vi "INI to JSON Test.vi"() -> ()   [LabVIEW 2017, in "JSONtext.lvlib"]
uses:
  JSONtext.lvlib
  support/quote and escape json string 2.vi
  <vilib>/JDP Science/JDP Science Common Utilities/JDP Utility.lvlib
panel:
  out "<JSON>":string
  out "String":string
  out "Array":string[](array[string])
  out "before substring":string
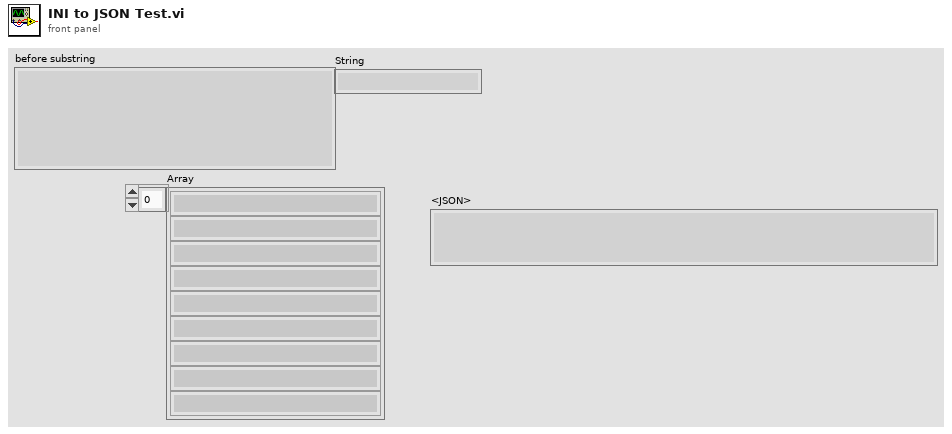
[diagram p1: front panel]
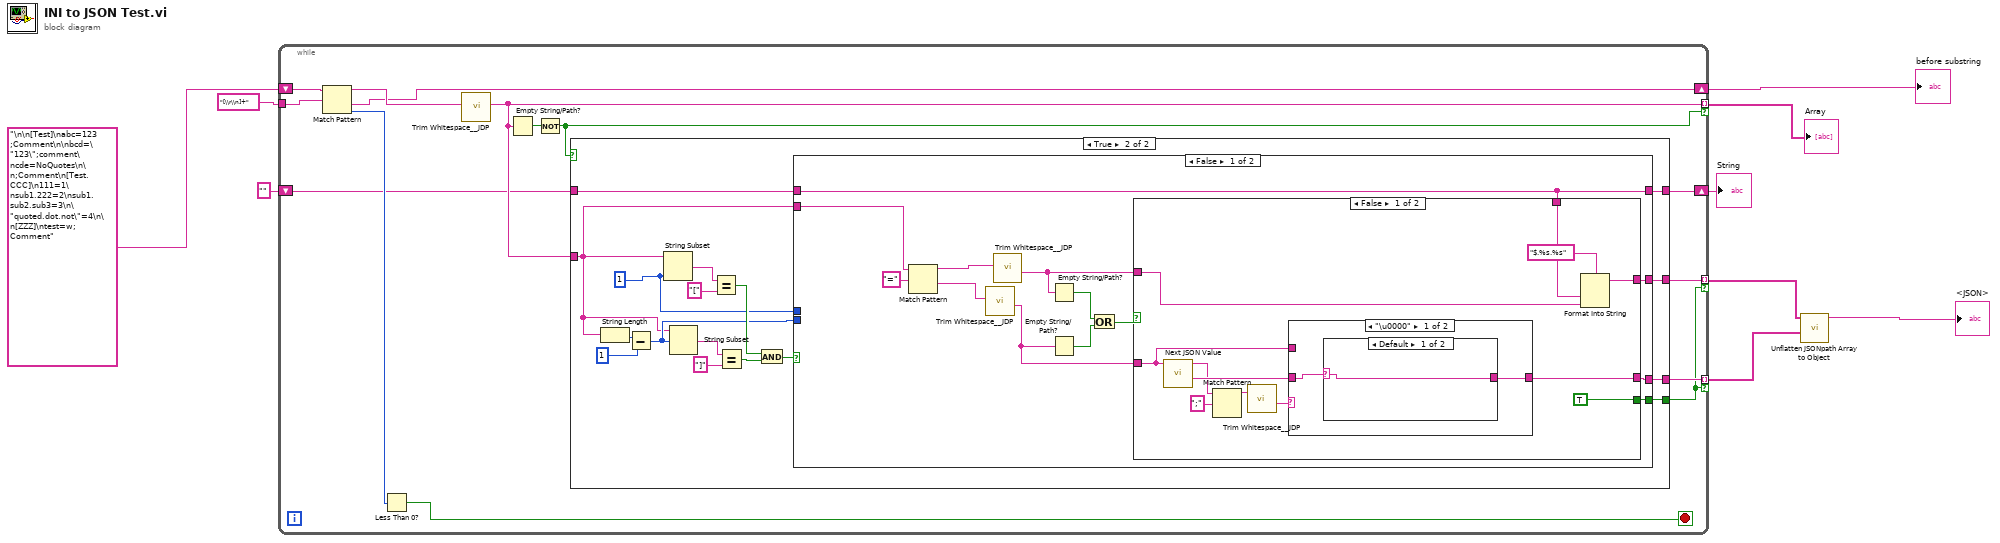
[diagram p0: block diagram]
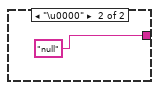
[diagram p3: hidden frame]
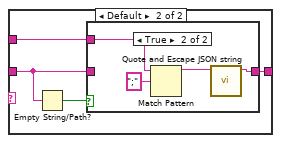
[diagram p4: hidden frame]
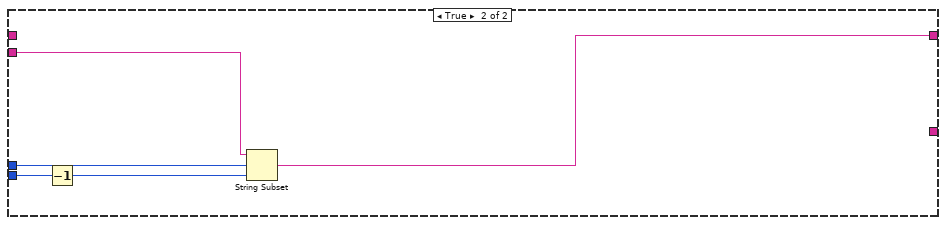
[diagram p7: hidden frame]
diagram:
  n1 = while {
    shift-right: [w20] -> w7
    shift-left: "\n\n[Test]\nabc=123 ;Comment\n\nbcd=\"123\";comment\ncde=NoQuotes\n\n;Comment\n[Test.CCC]\n111=1\nsub1.222=2\nsub1.sub2.sub3=3\n\"quoted.dot.not\"=4\n\n[ZZZ]\ntest=w; Comment" ("string") -> [w22]
    tunnel: "[\\r\\n]+" ("regular expression") -> [w23]
    tunnel: [w15] -> w6 mode=indexing if=w16
    shift-right: [w14] -> w4
    shift-left: "" -> [w13]
    tunnel: [w12] -> w2 mode=indexing if=w10
    tunnel: [w11] -> w3 mode=indexing if=w10
    stop <- w18 stop-if-true
    n2 = Match Pattern(string=w22, regular expression=w23) -> (before substring=w21:string, after substring=w20:string, offset past match=w19:i32)  [unwired: 1 in, 1 out]
    n3 = Less Than 0?(x=w19) -> (x < 0?=w18:bool)
    n4 = call <vilib>:"Trim Whitespace__JDP.vi"("String in"=w21) -> ("String out"=w15:string)  [unwired: 6 in]
    n5 = Empty String/Path?(string/path=w15) -> (empty?=w17:bool)
    n6 = Not(x=w17) -> (.not. x?=w16:bool)
    n7 = case shown="True" w16 {
      tunnel: w15 -> [_ w28]
      tunnel: [w24 w31] -> w14
      tunnel: w13 -> [w24 w29]
      tunnel: [_ w27] -> w12
      tunnel: [_ w26] -> w11
      tunnel: [_ w25] -> w10
      frame False {
      }
      frame True {
        w32 = 1 ("length (rest)")
        n8 = String Length(string=w28) -> (length=w37:i32)
        n9 = Subtract(x=w37, y=1) -> (x-y=w33:i32)
        n10 = String Subset(string=w28, length (rest)=w32) -> (substring=w41:string)  [unwired: 1 in]
        n11 = String Subset(string=w28, offset (0)=w33) -> (substring=w38:string)  [unwired: 1 in]
        n12 = Equal?(x=w41, y="[") -> (x = y?=w35:bool)
        n13 = Equal?(x=w38, y="]") -> (x = y?=w34:bool)
        n14 = And(x=w35, y=w34) -> (x .and. y?=w30:bool)
        n15 = case shown="False" w30 {
          tunnel: w33 -> [_ w84]
          tunnel: w32 -> [_ w83]
          tunnel: [w45 w82] -> w31
          tunnel: w29 -> [w45 _]
          tunnel: w28 -> [w54 w81]
          tunnel: [w44 _] -> w27
          tunnel: [w43 _] -> w26
          tunnel: [w42 _] -> w25
          frame False {
            n16 = Match Pattern(string=w54, regular expression="=") -> (before substring=w52:string, after substring=w51:string)  [unwired: 1 in, 2 out]
            n17 = call <vilib>:"Trim Whitespace__JDP.vi"("String in"=w51) -> ("String out"=w46:string)  [unwired: 6 in]
            n18 = call <vilib>:"Trim Whitespace__JDP.vi"("String in"=w52) -> ("String out"=w47:string)  [unwired: 6 in]
            n19 = Empty String/Path?(string/path=w47) -> (empty?=w50:bool)
            n20 = Empty String/Path?(string/path=w46) -> (empty?=w49:bool)
            n21 = Or(x=w50, y=w49) -> (x .or. y?=w48:bool)
            n22 = case shown="False" w48 {
              tunnel: w47 -> [w62 _]
              tunnel: w46 -> [w66 _]
              tunnel: w45 -> [w64 _]
              tunnel: [w63 _] -> w44
              tunnel: [w61 _] -> w43
              tunnel: [TRUE _] -> w42
              frame False {
                n23 = call "Next JSON Value.vi"("JSON"=w66) -> ("<JSON>"=w59:string, "Rest of Input String"=w57:string)  [unwired: 7 in, 2 out]
                n24 = Match Pattern(string=w57, regular expression=";") -> (before substring=w56:string)  [unwired: 1 in, 3 out]
                n25 = call <vilib>:"Trim Whitespace__JDP.vi"("String in"=w56) -> ("String out"=w55:string)  [unwired: 6 in]
                n26 = case shown="\"\"" w55 {
                  tunnel: w66 -> [_ w73]
                  tunnel: [w67 w72] -> w63
                  tunnel: w59 -> [w68 w71]
                  frame "\u0000" {
                    n27 = case shown="Default" w68 {
                      selector: w68 -> [w69 _]
                      tunnel: [w69 "null"] -> w67
                      frame Default {
                      }
                      frame "\u0000" {
                      }
                    }
                  }
                  frame Default {
                    n28 = Empty String/Path?(string/path=w71) -> (empty?=w74:bool)
                    n29 = case shown="True" w74 {
                      tunnel: w71 -> [w75 _]
                      tunnel: [w75 w79] -> w72
                      tunnel: w73 -> [_ w77]
                      frame False {
                      }
                      frame True {
                        n30 = Match Pattern(string=w77, regular expression=";") -> (before substring=w76:string)  [unwired: 1 in, 3 out]
                        n31 = call "Quote and Escape JSON string.vi"("Plain Text"=w76) -> ("<JSON>"=w79:string)  [unwired: 10 in]
                      }
                    }
                  }
                }
                n32 = Format Into String(format string="$.%s.%s", w64, w62) -> (resulting string=w61:string)  [unwired: 2 in, 1 out]
              }
              frame True {
              }
            }
          }
          frame True {
            n33 = Decrement(x=w84) -> (x-1=w80:i32)
            n34 = String Subset(string=w81, offset (0)=w83, length (rest)=w80) -> (substring=w82:string)
          }
        }
      }
    }
  }
  "before substring" <- w7
  "Array" <- w6
  "String" <- w4
  n35 = call "Unflatten JSONpath Array to Object.vi"("JSON Items"=w2, "$Paths"=w3) -> ("<JSON>"=→"<JSON>":string)  [unwired: 8 in, 1 out]
